vi "Substract_Array.vi"(7 "Substract Background":bool, 9 "Background":dbl[][](array[numeric]), 11 "Array":dbl[][](array[numeric])) -> (3 "Output Array":dbl[][](array[numeric]))   [LabVIEW 2013]
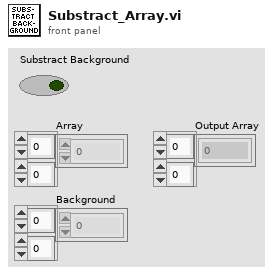
[diagram p1: front panel]
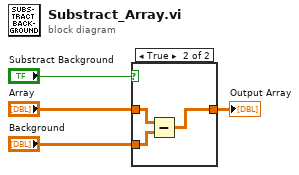
[diagram p0: block diagram]
diagram:
  n1 = case shown="True" "Substract Background" {
    tunnel: "Array" -> [w5 w8]
    tunnel: "Background" -> [_ w7]
    tunnel: [w5 w6] -> w1
    frame False {
    }
    frame True {
      n2 = Subtract(x=w8, y=w7) -> (x-y=w6:dbl[][])
    }
  }
  "Output Array" <- w1
